vi "GetCountOf.vi"(8 "error in (no error)":errorcluster, 10 "Countable":variant) -> (0 "error out":errorcluster, 2 "Count":i32)   [LabVIEW 2017, in "Transparent Assertions.lvlib" / "Constraints.lvlib" / "Count.lvclass"]
uses:
  Count.lvclass
  <vilib>/Utility/error.llb/Error Cluster From Error Code.vi
  <vilib>/ErrorRing/Error Ring.xnode
  <vilib>/Utility/Data Type/NI_Data Type.lvlib
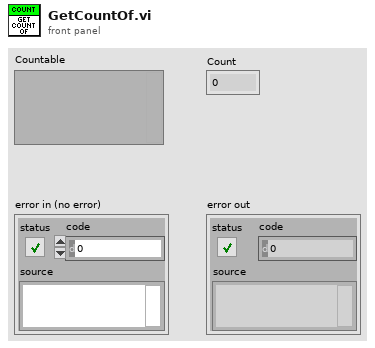
[diagram p1: front panel]
types:
  T1 = typedef "NI_Data Type.lvlib/Data Type.ctl" = enum8{"Invalid Type", "Void", "I8", "I16", "I32", "I64", "U8", "U16", "U32", "U64", "Single Float", "Double Float", "Extended Float", "Single Complex", "Double Complex", "Extended Complex", "Enum U8", "Enum U16", "Enum U32", "Enum U64", "Single Float With Unit", "Double Float With Unit", "Extended Float With Unit", "Single Complex with Unit", "Double Complex with Unit", "Extended Complex with Unit", "Boolean", "String", "Path", "Picture", "Tag", "Array", "Cluster", "Variant", "LV Variant", "Waveform", "Timestamp", "Digital Waveform", "Digital Data", "ExpressData", "Refnum", "External Data", "VI", "Poly VI", "LabVIEW Class Instance", "Fixed Point"}
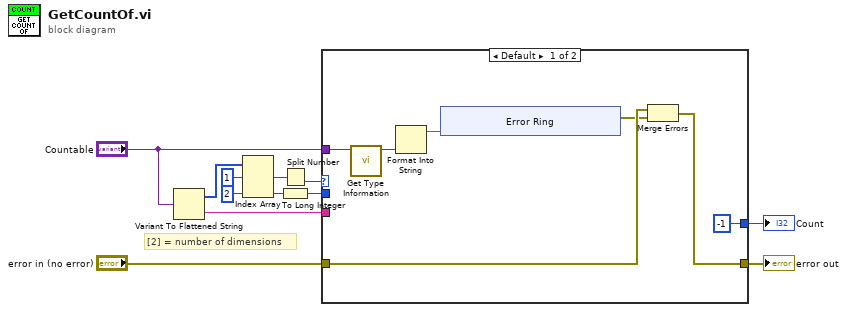
[diagram p0: block diagram]
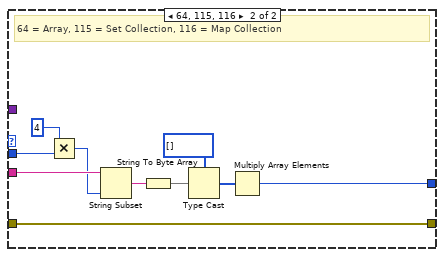
[diagram p2: hidden frame]
diagram:
  # "[2] = number of dimensions"
  n1 = Variant To Flattened String(Variant="Countable") -> (data string=w4:string, 1:w7:i16[])
  n2 = Index Array(array=w7, index #1=1 ("index"), index #3=2 ("index")) -> (element #1=w9:i16, element #3=w2:i16)  [unwired: 1 in, 1 out]
  n3 = To Long Integer(number=w2) -> (32bit integer=w1:i32)
  n4 = Split Number(x=w9) -> (lo(x)=w6:u8)  [unwired: 1 out]
  n5 = case shown="Default" w6 {
    tunnel: [-1 ("Count") w36] -> w12
    tunnel: [w17 w27] -> w11
    tunnel: "error in (no error)" -> [w19 w27]
    tunnel: "Countable" -> [w14 _]
    tunnel: w4 -> [_ w34]
    tunnel: w1 -> [_ w29]
    frame Default {
      n6 = call <vilib>:"Get Type Information.vi"("Variant"=w14) -> ("Type"=w13:T1)  [unwired: 6 in, 4 out]
      n7 = Format Into String(w13) -> (resulting string=w15:string)  [unwired: 3 in, 1 out]
      n8 = xnode "Error Ring"("parameter 0"=w15) -> ("error out"=w16:errorcluster)
      n9 = Merge Errors(w19, w16) -> (w17:errorcluster)
    }
    frame 64, 115, 116 {
      # "64 = Array, 115 = Set Collection, 116 = Map Collection"
      n10 = Multiply(x=4 ("length (rest)"), y=w29) -> (x*y=w28:i32)
      n11 = String Subset(string=w34, length (rest)=w28) -> (substring=w33:string)  [unwired: 1 in]
      n12 = String To Byte Array(string=w33) -> (unsigned byte array=w32:u8[])
      n13 = Type Cast(type=i32[] [], x=w32) -> (*(type *) &x=w35:i32[])
      n14 = Multiply Array Elements(1:w35) -> (0:w36:i32)
    }
  }
  "error out" <- w11
  "Count" <- w12
